vi "getCommandEvents.vi"(8 "error in (no error)":errorcluster, 11 "ConsoleViewer.lvclass in":refnum<class "ConsoleViewer.lvclass">) -> (0 "error out":errorcluster, 2 "Tools.lvlib:Interpreters.lvlib:CommandEvents.lvclass":refnum<class "CommandEvents.lvclass">, 3 "ConsoleViewer.lvclass out":refnum<class "ConsoleViewer.lvclass">)   [LabVIEW 2009, in "Views.lvlib" / "ConsoleViewer.lvclass"]
uses:
  ConsoleViewer.lvclass
  Tools/CommandProcessor/CommandEvents/CommandEvents.lvclass
  ConsoleViewer.lvclass/ConsoleViewer.ctl
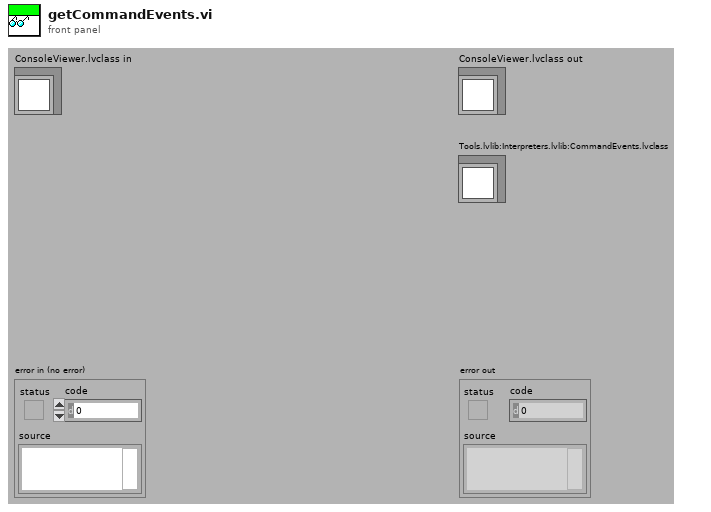
[diagram p1: front panel]
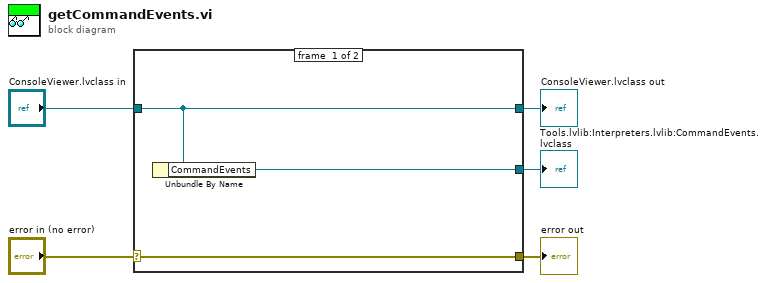
[diagram p0: block diagram]
diagram:
  n1 = case shown="No Error" "error in (no error)" {
    selector: "error in (no error)" -> [w8 w9]
    tunnel: [w8 w9] -> w4
    tunnel: [w7 w10] -> w2
    tunnel: "ConsoleViewer.lvclass in" -> [w7 w10]
    tunnel: [w6 _] -> w1
    frame #0 {
      n2 = Unbundle By Name(w7) -> ("CommandEvents"=w6:refnum<class "CommandEvents.lvclass">)
    }
    frame #1 {
    }
  }
  "error out" <- w4
  "ConsoleViewer.lvclass out" <- w2
  "Tools.lvlib:Interpreters.lvlib:CommandEvents.lvclass" <- w1
